vi "Detect Chassis.vi"(8 "error in":errorcluster, 10 "Controller in":refnum<class "Controller.lvclass">, 11 "Device in":refnum<class "SysCfg Device.lvclass">) -> (0 "error out":errorcluster, 2 "Controller out":refnum<class "Controller.lvclass">, 3 "Device out":refnum<class "SysCfg Device.lvclass">, 4 "Remote Chassis":refnum<class "Chassis.lvclass">[](array[class]), 6 "Local Chassis":refnum<class "Chassis.lvclass">)   [LabVIEW 2015, in "SMI.lvlib" / "Controller.lvclass"]
uses:
  Controller.lvclass
  SysCfg Device/SysCfg Device.lvclass
  Chassis/Chassis.lvclass
  SysCfg Device/SysCfg Device.lvclass/SysCfg Device.ctl
  Controller.lvclass/Controller.ctl
  SysCfg Device/Read SysCfg Session.vi
  SysCfg Device/Write SysCfg Session.vi
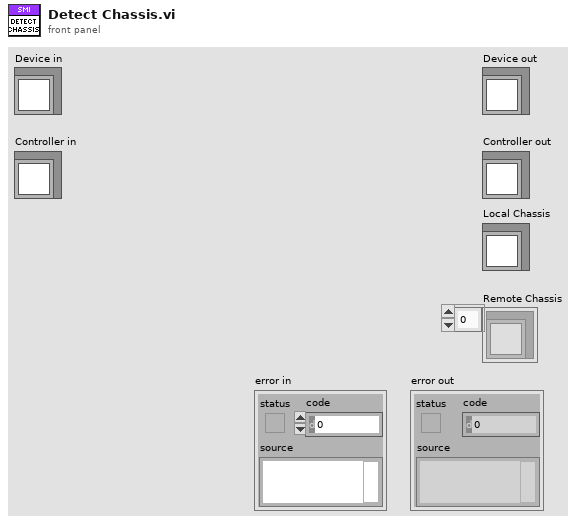
[diagram p1: front panel]
types:
  T1 = typedef "SMI.lvlib/Chassis.lvclass/ChassisInformation.ctl" = cluster{"Resource Name":string, "Vendor Name":string, "Product Name":string, "Product ID":u32, "Serial Number":string, "Number of Slots":i32}
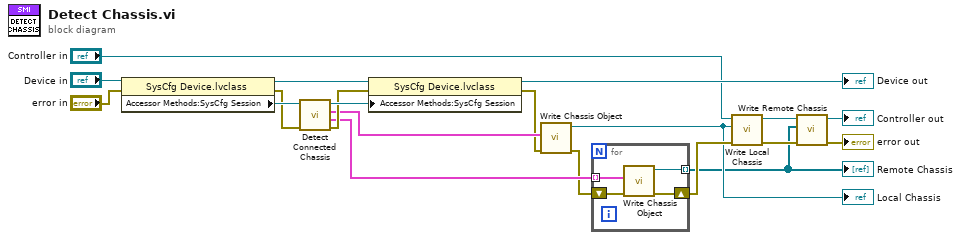
[diagram p0: block diagram]
diagram:
  n1 = property class="SysCfg Device.lvclass"(reference="Device in", error in="error in") -> (reference out=w16:refnum<class "SysCfg Device.lvclass">, error out=w19:errorcluster, "Accessor Methods:SysCfg Session"=w20:refnum<k21>)
  n2 = call "Detect Connected Chassis.vi"("error in"=w19, "SysCfg Session in"=w20) -> ("error out"=w14:errorcluster, "Remote Chassis"=w11:T1[], "Local Chassis"=w13:T1, "SysCfg Session out"=w15:refnum<k21>)  [unwired: 6 in]
  n3 = property class="SysCfg Device.lvclass"(reference=w16, error in=w14, "Accessor Methods:SysCfg Session"=w15) -> (reference out=→"Device out":refnum<class "SysCfg Device.lvclass">, error out=w12:errorcluster)
  n4 = call "Write Chassis Object.vi"("error in"=w12, "Chassis Information"=w13) -> ("error out"=w10:errorcluster, "Chassis out"=w2:refnum<class "Chassis.lvclass">)  [unwired: 8 in]
  "Local Chassis" <- w2
  n5 = for {
    tunnel: w11 -> [w24] mode=indexing
    shift-right: [w22] -> w3
    shift-left: w10 -> [w23]
    tunnel: [w21] -> w1 mode=indexing
    n6 = call "Write Chassis Object.vi"("error in"=w23, "Chassis Information"=w24) -> ("error out"=w22:errorcluster, "Chassis out"=w21:refnum<class "Chassis.lvclass">)  [unwired: 8 in]
  }
  "Remote Chassis" <- w1
  n7 = call "Write Local Chassis.vi"("error in"=w3, "Chassis in"=w2, "Controller in"="Controller in") -> ("error out"=w4:errorcluster, "Controller out"=w7:refnum<class "Controller.lvclass">)  [unwired: 7 in]
  n8 = call "Write Remote Chassis.vi"("error in"=w4, "Remote Chassis"=w1, "Controller in"=w7) -> ("error out"=→"error out":errorcluster, "Controller out"=→"Controller out":refnum<class "Controller.lvclass">)  [unwired: 7 in]
